vi "cursor_close.vi"(8 "error in (no error)":errorcluster, 11 "cursor":T1) -> (0 "error out":errorcluster)   [LabVIEW 2017, in "rethinkdb.lvlib"]
uses:
  rethinkdb.lvlib
  cursor_refnum.ctl
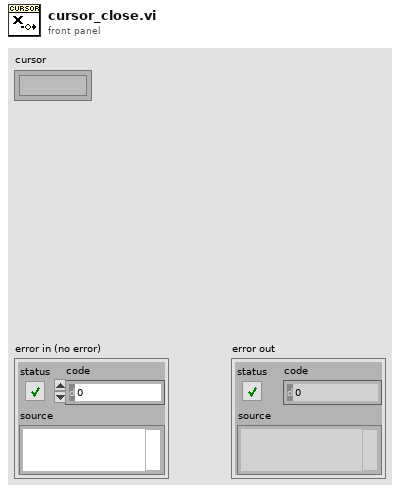
[diagram p1: front panel]
types:
  T1 = typedef "rethinkdb.lvlib/cursor_refnum.ctl" = refnum<k1>
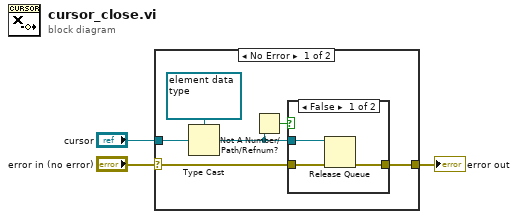
[diagram p0: block diagram]
diagram:
  n1 = case shown="No Error" "error in (no error)" {
    selector: "error in (no error)" -> [w7 w14]
    tunnel: "cursor" -> [w9 _]
    tunnel: [w6 w14] -> w2
    frame No Error {
      n2 = Type Cast(type=refnum<queue> refnum ("queue out"), x=w9) -> (*(type *) &x=w5:refnum<queue>)
      n3 = Not A Number/Path/Refnum?(number/path/refnum=w5) -> (NaN/Path/Refnum?=w4:bool)
      n4 = case shown="False" w4 {
        tunnel: w7 -> [w12 w13]
        tunnel: [w11 w13] -> w6
        tunnel: w5 -> [w10 _]
        frame False {
          n5 = Release Queue(queue=w10, error in (no error)=w12) -> (error out=w11:errorcluster)  [unwired: 1 in, 2 out]
        }
        frame True {
        }
      }
    }
    frame Error {
    }
  }
  "error out" <- w2
